vi "Stop Capture.vi"(3 "Error":string) -> (0 "Error":string)   [LabVIEW 2011, in "labvvis.lvlib"]
doc: "Returns the width and height of a LabVVIS image."
uses:
  <userlib>/labvvis/labvvis.lvlib
  labvvis.framework
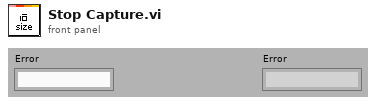
[diagram p1: front panel]
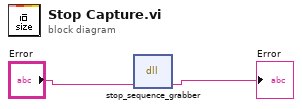
[diagram p0: block diagram]
diagram:
  n1 = dll-call lib="labvvis.framework" fn="stop_sequence_grabber"("error"="Error") -> ("error"=→"Error":string)  [unwired: 4 in, 2 out]
